vi "saveTestSTandSeq.vi"(0 "Engine reference":refnum<k7>, 5 "Sequence File Ref":refnum<k7>, 7 "pathString":string="c:\\temp\\testseq1.seq", 11 "error in":errorcluster) -> (4 "Engine reference(out)":refnum<k7>, 6 "Sequence File Ref(out)":refnum<k7>, 15 "error out":errorcluster)   [LabVIEW 2010]
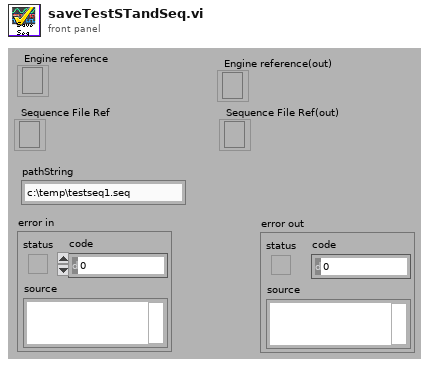
[diagram p1: front panel]
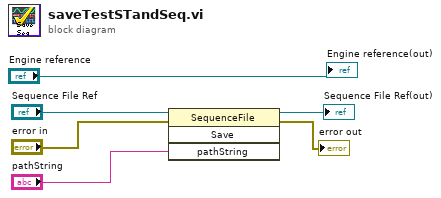
[diagram p0: block diagram]
diagram:
  n1 = invoke class="SequenceFile" method="Save"(reference="Sequence File Ref", error in="error in", "pathString"="pathString") -> (reference out=→"Sequence File Ref(out)":refnum<k7>, error out=→"error out":errorcluster)  [unwired: 1 in, 2 out]
  "Engine reference(out)" <- "Engine reference"
